vi "APC_9049_HRL_pegging.vi"(2 "exhaust pressure":dbl[](array[numeric]), 3 "Pcylfilt":dbl[](array[numeric])) -> (0 "Pressure pegging":dbl[][](graph), 1 "Pegged Pressure":dbl[](array[numeric]))   [LabVIEW 2020]
panel:
  in  "pegging interval length":i32=200
  in  "index for pegging":i32=6900
  in  "Graph?":bool
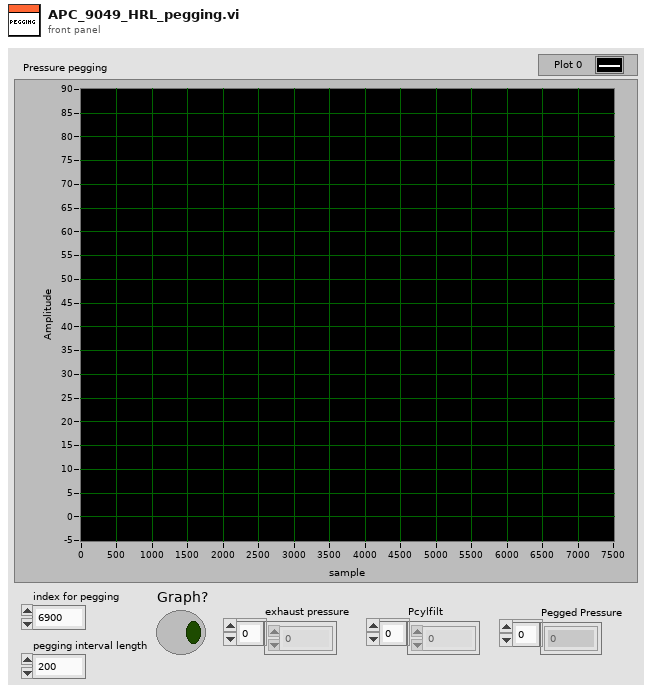
[diagram p1: front panel]
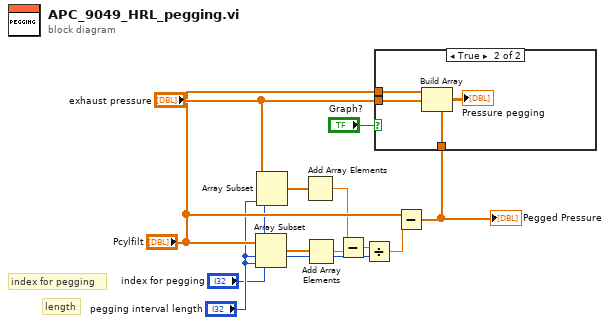
[diagram p0: block diagram]
diagram:
  # "length"
  # "index for pegging"
  n1 = Array Subset(array="Pcylfilt", index="index for pegging", length="pegging interval length") -> (w2:dbl[])
  n2 = Array Subset(array="exhaust pressure", index="index for pegging", length="pegging interval length") -> (w4:dbl[])
  n3 = Add Array Elements(numeric array=w4) -> (sum=w6:dbl)
  n4 = Add Array Elements(numeric array=w2) -> (sum=w5:dbl)
  n5 = Subtract(x=w5, y=w6) -> (x-y=w7:dbl)
  n6 = Divide(x=w7, y="pegging interval length") -> (x/y=w9:dbl)
  n7 = Subtract(x="Pcylfilt", y=w9) -> (x-y=w11:dbl[])
  "Pegged Pressure" <- w11
  n8 = case shown="True" "Graph?" {
    tunnel: "exhaust pressure" -> [_ w16]
    tunnel: w11 -> [_ w15]
    tunnel: "Pcylfilt" -> [_ w14]
    frame False {
    }
    frame True {
      n9 = Build Array(w14, w16, w15) -> (→"Pressure pegging":dbl[][])
    }
  }
